vi "Get IPC State.vi"(10 "reset":bool, 11 "index":u16) -> ()   [LabVIEW 2025, in "ExtremelyEpicImagerIPC2.lvlib"]
doc: "IMAGERIPC_API USHORT WINAPI GetIPCState(WORD index, bool reset);"
uses:
  ExtremelyEpicImagerIPC2.lvlib
  ImagerIPC2.dll
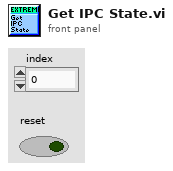
[diagram p1: front panel]
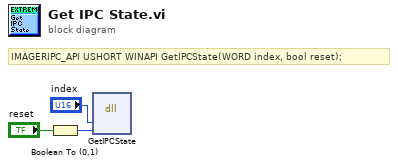
[diagram p0: block diagram]
diagram:
  # "IMAGERIPC_API USHORT WINAPI GetIPCState(WORD index, bool reset);"
  n1 = Boolean To (0,1)(Boolean="reset") -> (0, 1=w1:i16)
  n2 = dll-call lib="C:/Users/mayhe/OneDrive/Documents/GitHub/In-situ-monitoring-of-powder-bed-fusion-additive-manufacturing/system_development/Orichalcum/v0.2/Software_design/thermal-camera/VI/Connect SDK/ImagerIPC2.*" fn="GetIPCState"("index"="index", "reset"=w1) -> ()  [unwired: 6 in, 2 out]
